vi "read_symbols_from_project_item.vi"(8 "error in (no error)":errorcluster, 11 "ProjectItem in":refnum<vi>) -> (0 "error out":errorcluster, 1 "CCSymbols":map{string, string}(c390), 2 "CCSymbols out":string, 3 "ProjectItem out":refnum<vi>)   [LabVIEW 2019, in "Conditional Disable Build Actions.lvlib"]
uses:
  Conditional Disable Build Actions.lvlib
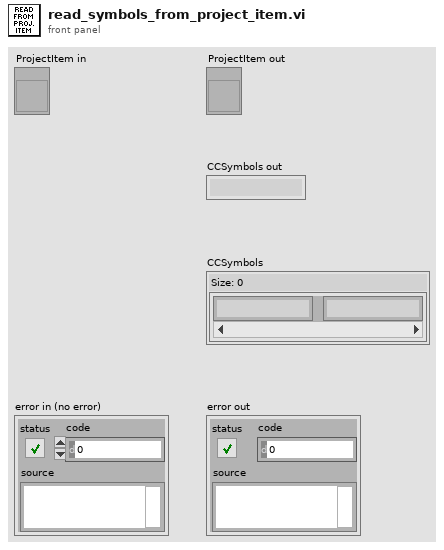
[diagram p1: front panel]
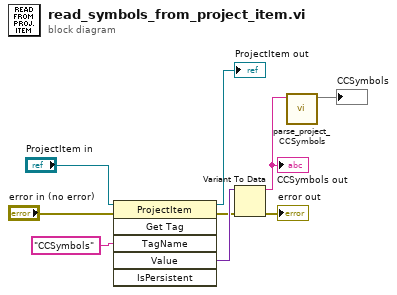
[diagram p0: block diagram]
diagram:
  n1 = invoke class="ProjectItem" method="Get Tag"(reference="ProjectItem in", error in="error in (no error)", "TagName"="CCSymbols" ("Tag Name")) -> (reference out=→"ProjectItem out":refnum<vi>, error out=w2:errorcluster, "Value"=w6:variant)  [unwired: 3 in, 3 out]
  n2 = Variant To Data(error in=w2, Variant=w6) -> (data=w8:string, error out=→"error out":errorcluster)  [unwired: 1 in]
  "CCSymbols out" <- w8
  n3 = call "parse_project_CCSymbols.vi"("CCSymbols from Project"=w8) -> ("CCSymbols"=→"CCSymbols":map{string, string})  [unwired: 10 in]
